vi "Flush Data to Log File.vi"(8 "error in (no error)":errorcluster, 10 "Data Queue":refnum<queue>, 11 "Logging Configuration":T1) -> (0 "error out":errorcluster)   [LabVIEW 2022 SP3, in "Logging.lvlib"]
doc: "Flush the data queue of any pending data and write it to the log file. Close the TDMS file reference."
uses:
  Logging.lvlib
  Logging Configuration.ctl
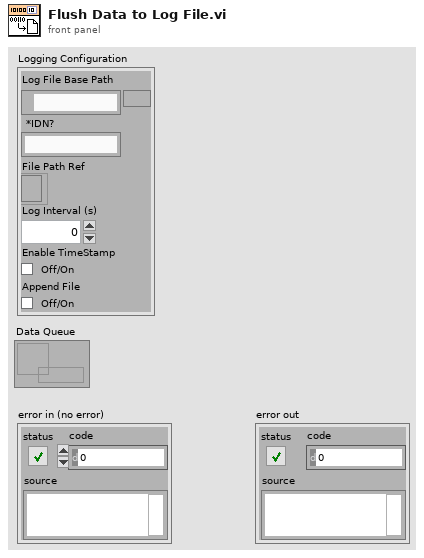
[diagram p1: front panel]
types:
  T1 = typedef "Logging.lvlib/Logging Configuration.ctl" = cluster{"Log File Base Path":path, "*IDN?":string, "File Path Ref":refnum<file>, "Log Interval (s)":dbl, "Enable TimeStamp":bool, "Append File":bool}
  T2 = enum16{"open", "replace", "create", "open or create", "replace or create", "replace or create with confirmation"}
  T3 = cluster{"Numeric":dbl, "Numeric":dbl, "Numeric":dbl, timestamp}[]
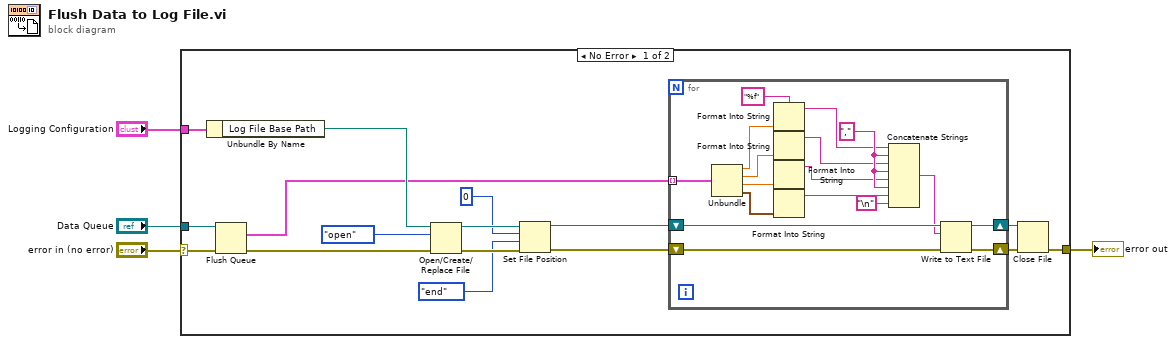
[diagram p0: block diagram]
diagram:
  n1 = case shown="No Error" "error in (no error)" {
    selector: "error in (no error)" -> [w11 w38]
    tunnel: "Data Queue" -> [w12 _]
    tunnel: "Logging Configuration" -> [w13 _]
    tunnel: [w8 w38] -> w3
    frame No Error {
      n2 = Unbundle By Name(w13) -> ("Log File Base Path"=w15:path)
      n3 = Flush Queue(queue=w12, error in (no error)=w11) -> (remaining elements=w10:T3, error out=w14:errorcluster)  [unwired: 1 out]
      n4 = Open/Create/Replace File(file path (use dialog)=w15, error in=w14, operation (0:open)=T2."open") -> (refnum out=w19:refnum<file>, error out=w18:errorcluster)  [unwired: 3 in, 1 out]
      n5 = Set File Position(offset (in bytes) (0)=i64 0, refnum=w19, from (0:start)=enum16{"start", "end", "current"}."end", error in=w18) -> (refnum out=w6:refnum<file>, error out=w9:errorcluster)
      n6 = for {
        tunnel: w10 -> [w26] mode=indexing
        shift-right: [w24] -> w7
        shift-left: w9 -> [w25]
        shift-right: [w22] -> w5
        shift-left: w6 -> [w23]
        w34 = ","
        w30 = "%f"
        n7 = Unbundle(w26) -> ("Numeric"=w35:dbl, "Numeric"=w36:dbl, "Numeric"=w37:dbl, w29:timestamp)
        n8 = Format Into String(format string=w30, w35) -> (resulting string=w33:string)  [unwired: 2 in, 1 out]
        n9 = Format Into String(format string=w30, w36) -> (resulting string=w32:string)  [unwired: 2 in, 1 out]
        n10 = Format Into String(format string=w30, w37) -> (resulting string=w31:string)  [unwired: 2 in, 1 out]
        n11 = Format Into String(w29) -> (resulting string=w28:string)  [unwired: 3 in, 1 out]
        n12 = Concatenate Strings(w33, w34, w32, w34, w31, w34, w28, "\n") -> (w21:string)
        n13 = Write to Text File(file (use dialog)=w23, text=w21, error in=w25) -> (refnum out=w22:refnum<file>, error out=w24:errorcluster)  [unwired: 1 in, 1 out]
      }
      n14 = Close File(refnum=w5, error in=w7) -> (error out=w8:errorcluster)  [unwired: 1 out]
    }
    frame Error {
    }
  }
  "error out" <- w3
